vi "Volume ROI entry user dialogue handler.vi"(7 "Center around clicked pixel (F)":bool, 8 "error in (no error)":errorcluster, 11 "New coordinates":i32[](array[numeric])) -> (0 "error IO":errorcluster, 1 "Cancelled":bool, 3 "ROIs Info []":T1[](array[typedef]) {"Zoom" min=1.0 max=10.0 step=0.10000000149011612})   [LabVIEW 2017]
uses:
  Typedefs/ROI spec.ctl
  Typedefs/ROI ID Enum.ctl
  ROI Entry screen/Globals/gl_ROI Entry UI globals.vi
panel:
  out "Modified coordinates":i32[](array[numeric])
  # "Tick the box below if you want to specify a volume from the rectangular shaped you have drawn and enter select the two z--planes between which the volume should be created."
  # "X1\nY1\nX2\nY2"
  # "X1\nY1\nX2\nY2"
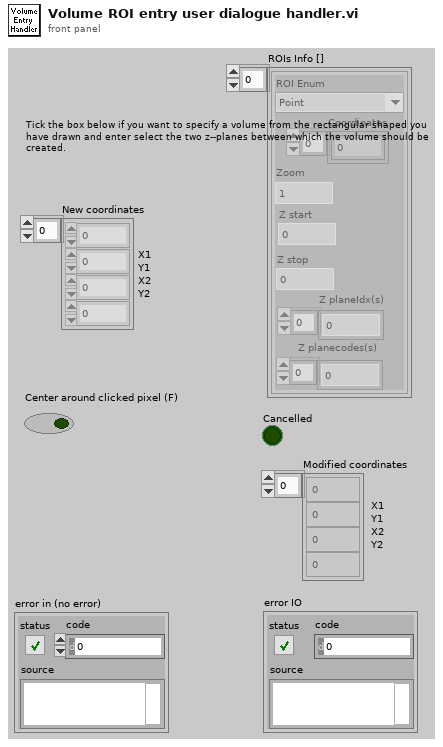
[diagram p1: front panel]
types:
  T1 = typedef "ROI spec.ctl" = cluster{"Coordinates":i32[], "Zoom":dbl, "ROI Enum":T2, "Z planeIdx(s)":i32[], "Z planecodes(s)":u8[], "Z start":dbl, "Z stop":dbl}
  T2 = typedef "ROI ID Enum.ctl" = enum16{"Point", "MiniScan", "Comp. MiniScan", "Rectangle", "Comp. volume", "Arb. plane point", "None"}
  T3 = typedef "ROI entry screen ctrl refs cluster.ctl" = cluster{"Done button":refnum<vi>, "Imaging button":refnum<vi>, "Acquisition button":refnum<vi>, "POI dwell time (us)":refnum<vi>, "Scan dwell time per pixel (us)":refnum<vi>, "# of planes":refnum<vi>, "Zoom Ctrl":refnum<vi>, "Equal size":refnum<vi>, "Channel":refnum<vi>, "Image Display":refnum<vi>, "Z-Plane Selector":refnum<vi>, "Number of lines left":refnum<vi>, "Z-stack folder path":refnum<vi>, "POI Density":refnum<vi>, "Arb Plane Entry":refnum<vi>, "Whole plane":refnum<vi>, "Clear Last":refnum<vi>, "Clear All":refnum<vi>, "Trial Length (sec)":refnum<vi>, "Palette Type":refnum<vi>, "Intensity slider":refnum<vi>, "# POI":refnum<vi>, "Max Z Proj":refnum<vi>, "Zplane ind":refnum<vi>, "Wavelength (nm)":refnum<vi>, "Number of Trials":refnum<vi>, "Funct stim.trig.enable":refnum<vi>, "Funct stim.trig.delay (s)":refnum<vi>, "Line Mode":refnum<vi>, "Step size (µm)":refnum<vi>, "ROI move mode":refnum<vi>, "Cool-down time (s)":refnum<vi>, "Enable cool-down time":refnum<vi>, "Motor Z ind. (um)":refnum<vi>, "AOL Z ind. (um)":refnum<vi>, "Load Reference Image":refnum<vi>}
  T4 = typedef "ROI input mode.ctl" = enum16{"Unspecified", "Point-Line-Plane", "Volume"}
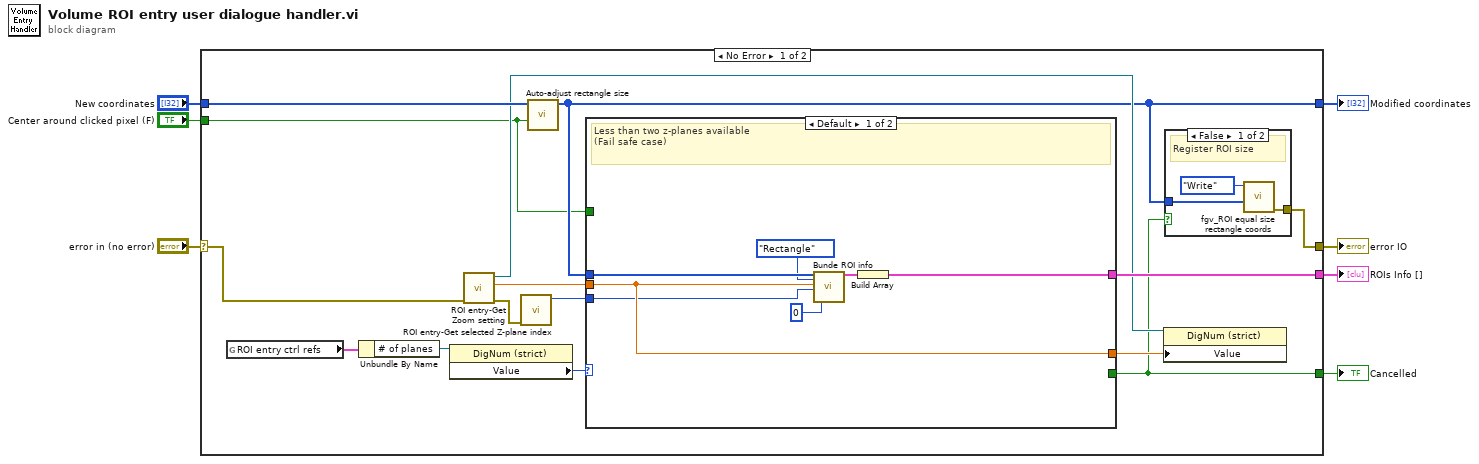
[diagram p0: block diagram]
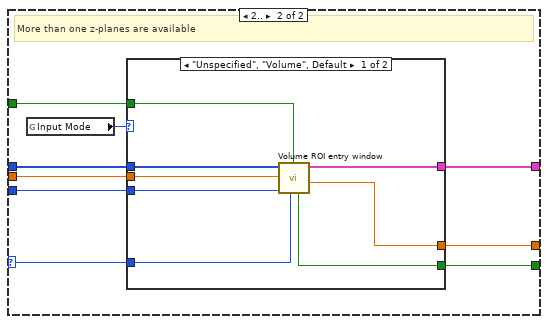
[diagram p3: hidden frame]
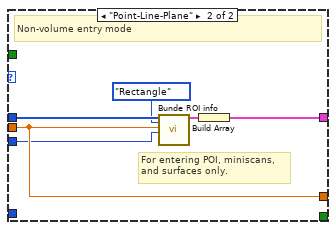
[diagram p4: hidden frame]
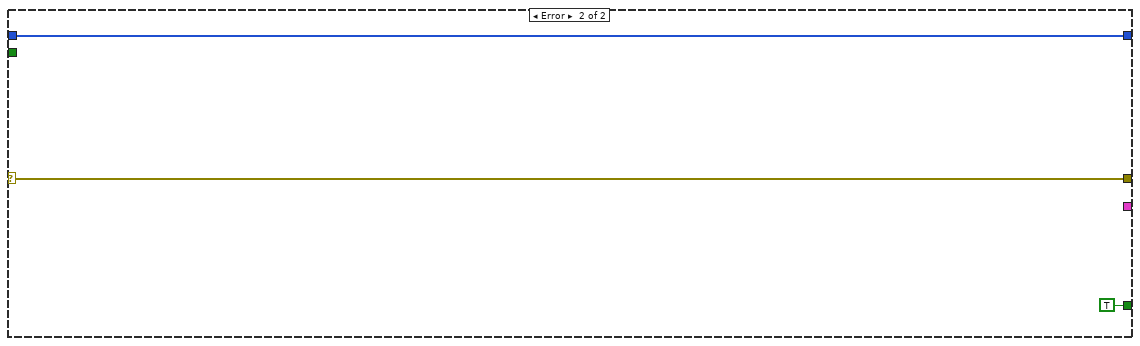
[diagram p5: hidden frame]
diagram:
  n1 = case shown="No Error" "error in (no error)" {
    selector: "error in (no error)" -> [w9 w58]
    tunnel: [w22 _] -> w7
    tunnel: "New coordinates" -> [w21 w56]
    tunnel: [w13 w56] -> w5
    tunnel: [w12 TRUE ("Cancelled")] -> w4
    tunnel: [w10 w58] -> w2
    tunnel: "Center around clicked pixel (F)" -> [w8 _]
    frame No Error {
      n2 = global read "gl_ROI Entry UI globals.vi" "ROI entry ctrl refs"() -> (w19:T3)
      n3 = Unbundle By Name(w19) -> ("# of planes"=w20:refnum<vi>)
      n4 = property class="DigNum (strict)"(reference=w20) -> ("Value"=w18:i32)  [unwired: 1 in, 2 out]
      n5 = call "ROI entry-Get Zoom setting.vi"("error in (no error)"=w9) -> ("error out"=w11:errorcluster, "Zoom Value"=w16:dbl, "Zoom control ref"=w15:refnum<vi>)  [unwired: 8 in]
      n6 = call "ROI entry-Get selected Z-plane index.vi"("error in (no error)"=w11) -> ("Z-plane selector (index)"=w14:i32)  [unwired: 9 in, 1 out]
      n7 = call "Auto-adjust rectangle size.vi"("Center around clicked pixel (F)"=w8, "New Coordinates"=w21) -> ("Modified coordinates"=w13:i32[])  [unwired: 9 in]
      n8 = case shown="Default" w18 {
        selector: w18 -> [_ w38]
        tunnel: [w32 w39] -> w22
        tunnel: w13 -> [w31 w41]
        tunnel: w14 -> [w27 w40]
        tunnel: [_ w37] -> w12
        tunnel: w16 -> [w29 w35]
        tunnel: [w29 w34] -> w17
        tunnel: w8 -> [_ w33]
        frame Default {
          # "Less than two z-planes available\n(Fail safe case)"
          n9 = call "Bunde ROI info.vi"("ROI Coordinates"=w31, "ROI Enum"=ROI_ID_Enum."Rectangle", "Zoom"=w29, "ZplaneIndex"=w27, "Zplanecode"=u8 0) -> ("ROI Info"=w30:T1)  [unwired: 14 in]
          n10 = Build Array(w30) -> (w32:T1[])
        }
        frame 2.. {
          # "More than one z-planes are available"
          n11 = global read "gl_ROI Entry UI globals.vi" "Input Mode"() -> (w36:T4)
          n12 = case shown="\"Unspecified\", \"Volume\", Default" w36 {
            tunnel: w41 -> [w49 w54]
            tunnel: w40 -> [w48 w50]
            tunnel: [w47 w55] -> w39
            tunnel: w38 -> [w46 _]
            tunnel: [w45 _] -> w37
            tunnel: w35 -> [w44 w52]
            tunnel: [w43 w52] -> w34
            tunnel: w33 -> [w42 _]
            frame "Unspecified", "Volume", Default {
              n13 = call "Volume ROI entry window.vi"("# of planes"=w46, "Do not initialise selector values"=w42, "ZplaneIndex (zero based)"=w48, "Zoom (in)"=w44, "Coordinates"=w49) -> ("Zoom (out)"=w43:dbl, "ROIs Info []"=w47:T1[], "Cancelled"=w45:bool)  [unwired: 4 in]
            }
            frame "Point-Line-Plane" {
              # "For entering POI, miniscans,\nand surfaces only."
              # "Non-volume entry mode"
              n14 = call "Bunde ROI info.vi"("ROI Coordinates"=w54, "ROI Enum"=ROI_ID_Enum."Rectangle", "Zoom"=w52, "ZplaneIndex"=w50) -> ("ROI Info"=w53:T1)  [unwired: 15 in]
              n15 = Build Array(w53) -> (w55:T1[])
            }
          }
        }
      }
      n16 = property class="DigNum (strict)"(reference=w15, "Value"=w17) -> ()  [unwired: 1 in, 2 out]
      n17 = case shown="False" w12 {
        tunnel: w13 -> [w25 _]
        tunnel: [w23 _] -> w10
        frame False {
          # "Register ROI size"
          n18 = call "fgv_ROI equal size rectangle coords.vi"("New Rectangle Coordinates"=w25, "Function"=enum16{"Intialize", "Write", "Read", "Clear"}."Write") -> ("error out"=w23:errorcluster)  [unwired: 8 in, 1 out]
        }
        frame True {
        }
      }
    }
    frame Error {
    }
  }
  "ROIs Info []" <- w7
  "Cancelled" <- w4
  "Modified coordinates" <- w5
  "error IO" <- w2
